vi "GetVariableField.vi"(10 "Field":refnum<k24>, 11 "error in (no error)":errorcluster) -> (2 "Field cluster":T1, 3 "error out":errorcluster)   [LabVIEW 2018, in "UnderAutomation.Fanuc.lvlib"]
uses:
  UnderAutomation.Fanuc.lvlib
  C:/Users/fg/Documents/Fanuc.vi/LabVIEW_2024/UnderAutomation.Fanuc/lib/UnderAutomation.Fanuc.dll
  LabVIEW_2024/UnderAutomation.Fanuc/lib/UnderAutomation.Fanuc.dll
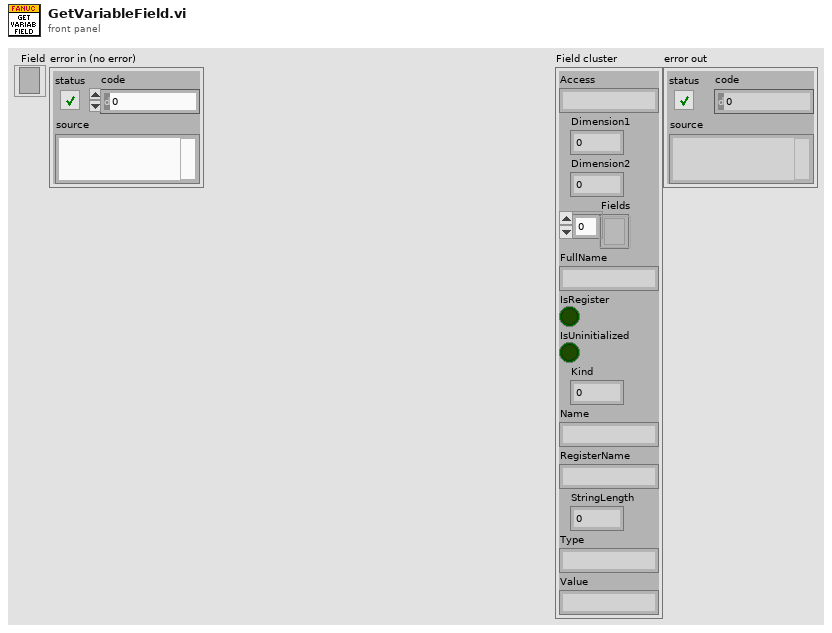
[diagram p1: front panel]
types:
  T1 = cluster{"Access":string, "Dimension1":i32, "Dimension2":i32, "Fields":refnum<k24>[], "FullName":string, "IsRegister":bool, "IsUninitialized":bool, "Kind":i32, "Name":string, "RegisterName":string, "StringLength":i32, "Type":string, "Value":string}
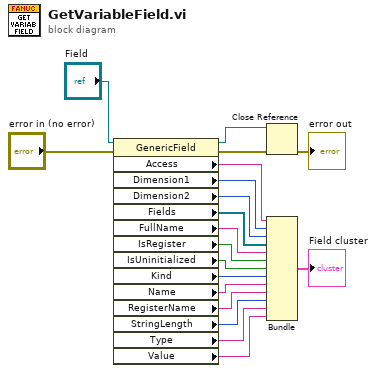
[diagram p0: block diagram]
diagram:
  n1 = property class="GenericField"(reference="Field", error in="error in (no error)") -> (reference out=w1:refnum<k24>, error out=w3:errorcluster, "Access"=w18:string, "Dimension1"=w17:i32, "Dimension2"=w16:i32, "Fields"=w15:refnum<k24>[], "FullName"=w14:string, "IsRegister"=w13:bool, "IsUninitialized"=w12:bool, "Kind"=w11:i32, "Name"=w10:string, "RegisterName"=w9:string, "StringLength"=w8:i32, "Type"=w7:string, "Value"=w6:string)
  n2 = Close Reference(reference=w1, error in (no error)=w3) -> (error out=→"error out":errorcluster)
  n3 = Bundle("Access"=w18, "Dimension1"=w17, "Dimension2"=w16, "Fields"=w15, "FullName"=w14, "IsRegister"=w13, "IsUninitialized"=w12, "Kind"=w11, "Name"=w10, "RegisterName"=w9, "StringLength"=w8, "Type"=w7, "Value"=w6) -> (→"Field cluster":T1)  [unwired: 1 in]
